vi "Feeding_OPEN_DOOR_ON_SCAN.vi"(7 "CYCLE DATA IN":T1, 8 "error in (no error)":errorcluster, 11 "raw scan code":string) -> (0 "error out":errorcluster, 2 "search valid ?":bool, 5 "CYCLE DATA OUT":T1)   [LabVIEW 2017]
uses:
  Controls/Feed_Cyc_Data.ctl
  <vilib>/Utility/file.llb/Read Delimited Spreadsheet (string).vi
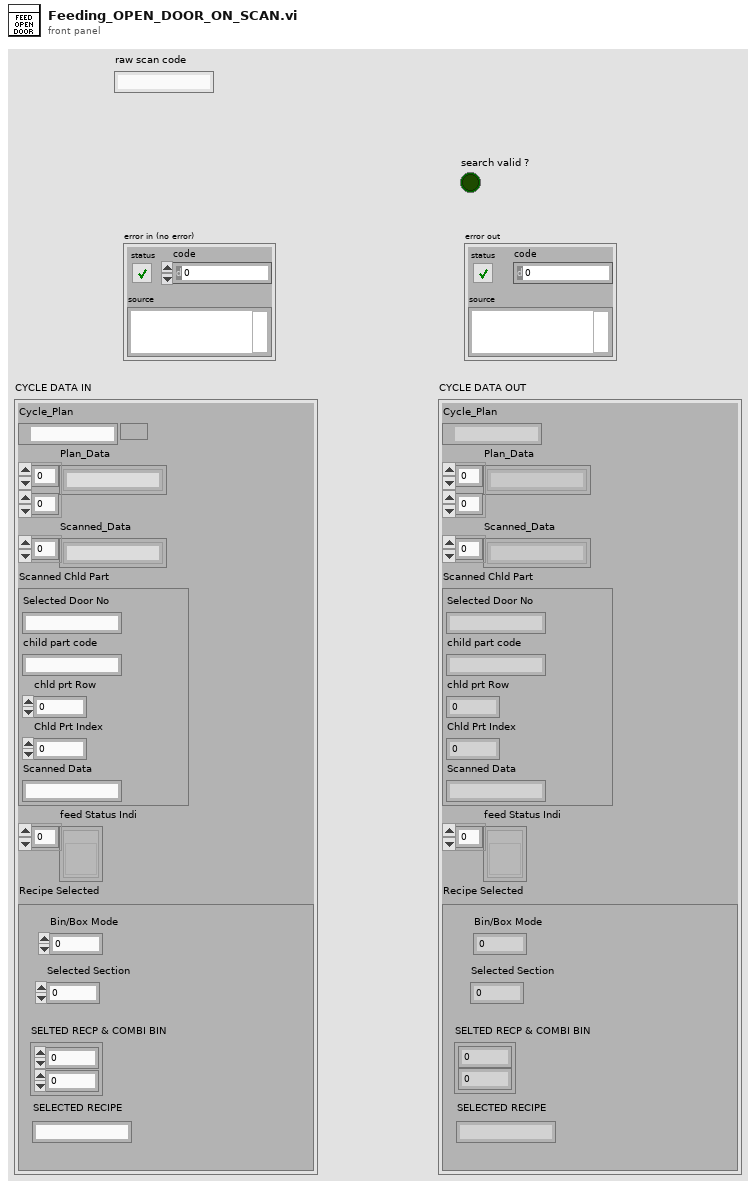
[diagram p1: front panel]
types:
  T1 = typedef "Feed_Cyc_Data.ctl" = cluster{"Cycle_Plan":path, "Plan_Data":string[][], "Scanned_Data":string[], "Scanned Chld Part":cluster{"Selected Door No":string, "child part code":string, "chld prt Row":i32, "Chld Prt Index":i32, "Scanned Data":string}, "feed Status Indi":refnum<vi>[], "Recipe Selected":cluster{"Bin/Box Mode":i32, "Selected Section":i32, "SELTED RECP & COMBI BIN":cluster{i32, i32}, "SELECTED RECIPE":string}}
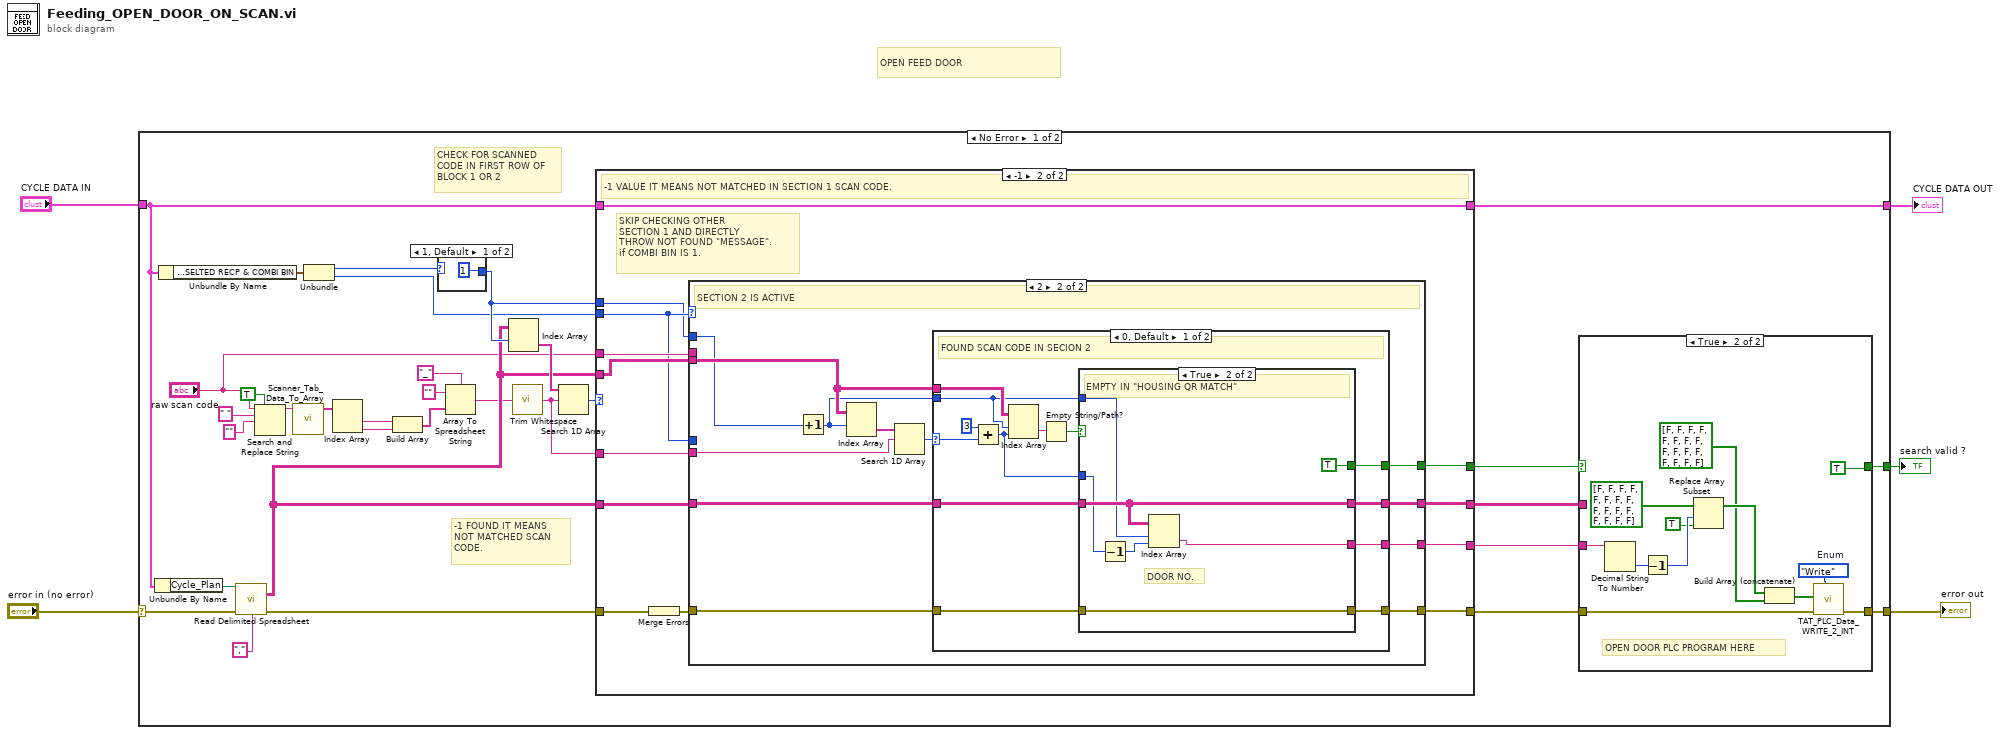
[diagram p0: block diagram]
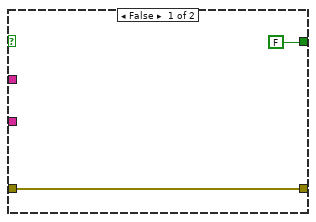
[diagram p2: hidden frame]
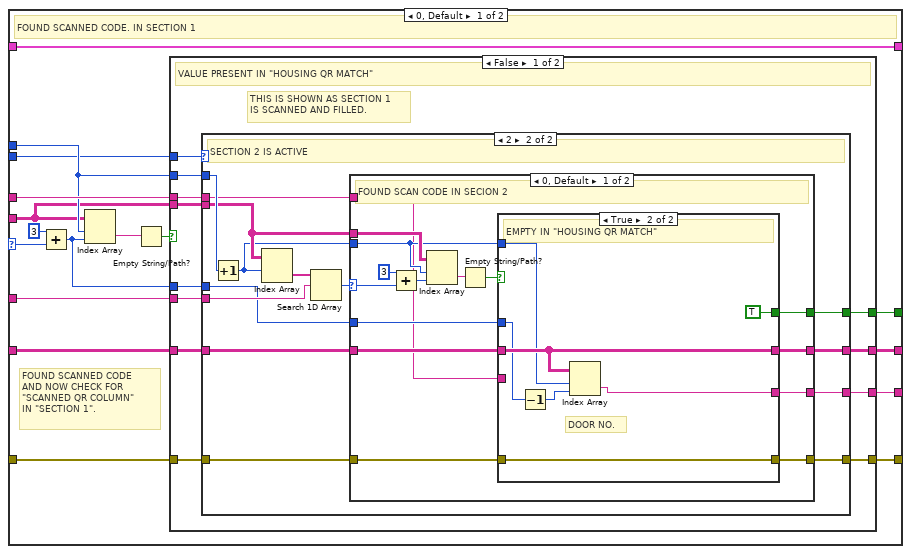
[diagram p3: hidden frame]
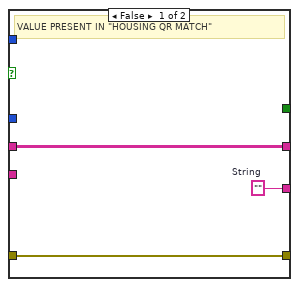
[diagram p5: hidden frame]
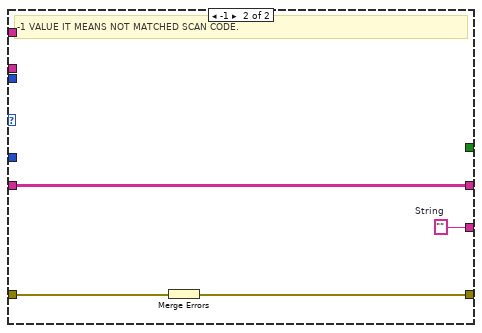
[diagram p6: hidden frame]
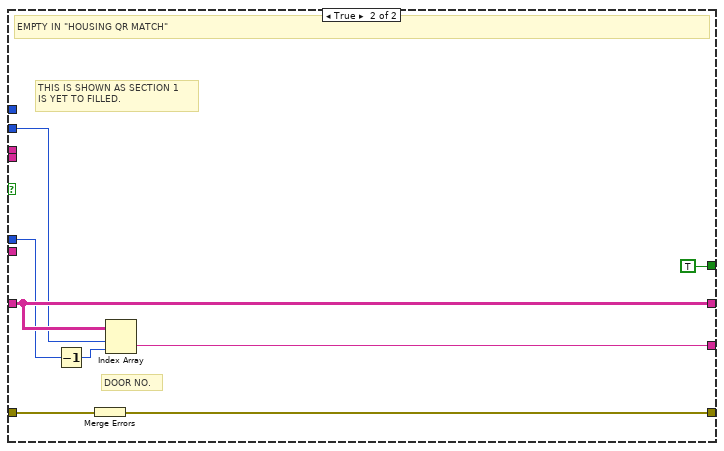
[diagram p7: hidden frame]
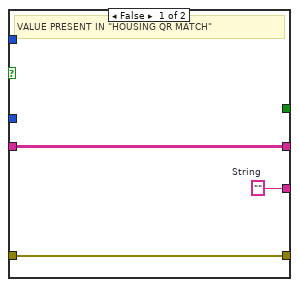
[diagram p9: hidden frame]
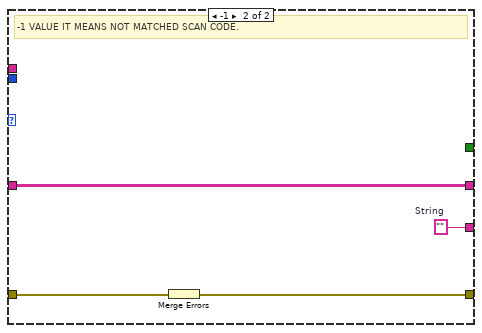
[diagram p10: hidden frame]
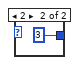
[diagram p11: hidden frame]
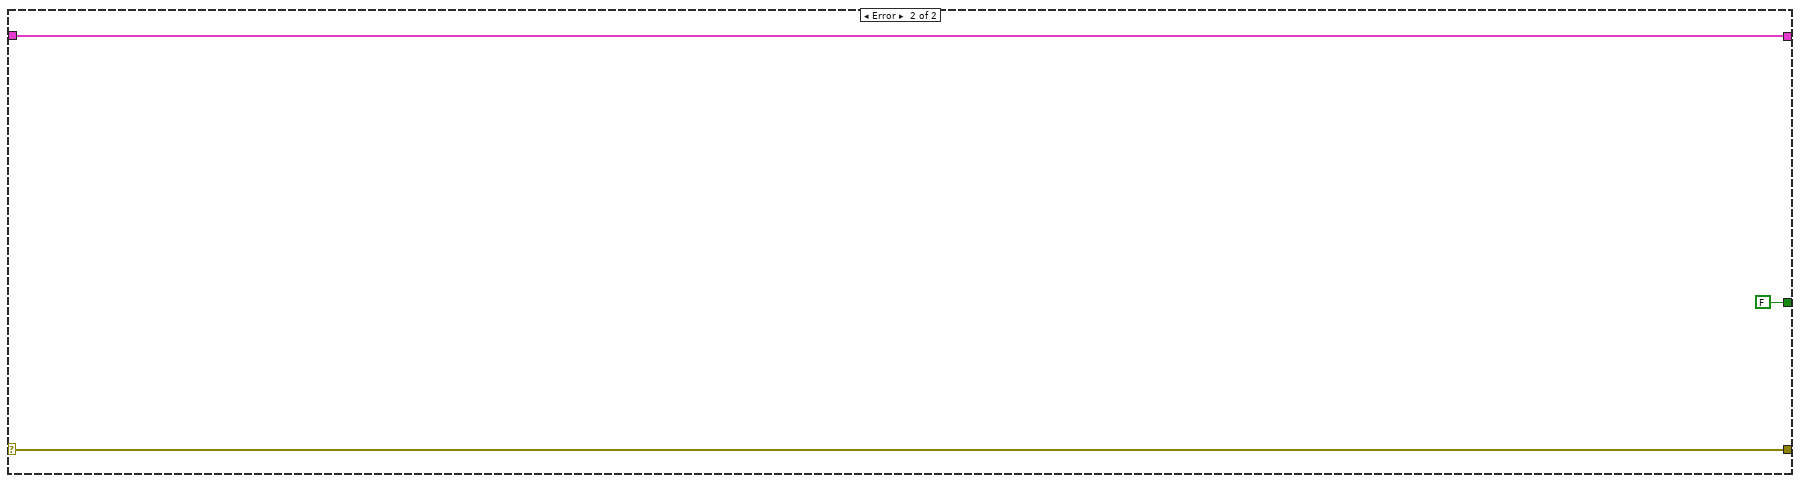
[diagram p12: hidden frame]
diagram:
  # "OPEN FEED DOOR"
  n1 = case shown="No Error" "error in (no error)" {
    selector: "error in (no error)" -> [w34 w192]
    tunnel: [w18 w192] -> w4
    tunnel: [w16 w191] -> w2
    tunnel: "CYCLE DATA IN" -> [w23 w191]
    tunnel: [w8 FALSE] -> w1
    frame No Error {
      # "-1 FOUND IT MEANS\nNOT MATCHED SCAN\nCODE."
      # "CHECK FOR SCANNED\nCODE IN FIRST ROW OF\nBLOCK 1 OR 2"
      n2 = Unbundle By Name(w23) -> ("Cycle_Plan"=w35:path)
      n3 = Unbundle By Name(w23) -> ("Recipe Selected.SELTED RECP & COMBI BIN"=w32:cluster{i32, i32})
      n4 = call-poly <vilib>:"Read Delimited Spreadsheet.vi"("file path (dialog if empty)"=w35, "error in (no error)"=w34, "delimiter (\\t)"=",") -> ("all rows"=w20:string[][], "error out"=w33:errorcluster)  [unwired: 7 in, 4 out]
      n5 = Search and Replace String(replace all?=TRUE, input string="raw scan code", search string=" ", replace string="") -> (result string=w30:string)  [unwired: 4 in, 3 out]
      n6 = call "Scanner_Tab_Data_To_Array.vi"("Scanner Data"=w30) -> ("Array"=w14:string[])  [unwired: 10 in]
      n7 = Unbundle(w32) -> (w31:i32, w19:i32)
      n8 = Index Array(array=w14) -> (element #1=w13:string, element #2=w12:string)  [unwired: 2 in]
      n9 = Build Array(w13, w12) -> (w11:string[])
      n10 = case shown="1, Default" w31 {
        tunnel: [1 3] -> w21
        frame 1, Default {
        }
        frame 2 {
        }
      }
      n11 = Array To Spreadsheet String(delimiter (Tab)="_", array=w11, 3:"") -> (spreadsheet string=w10:string)
      n12 = Index Array(array=w20, index (row)=w21) -> (element=w24:string[])  [unwired: 1 in]
      n13 = call <vilib>:"Trim Whitespace.vi"("string"=w10) -> ("trimmed string"=w6:string)  [unwired: 1 in]
      n14 = Search 1D Array(1D array=w24, element=w6) -> (index of element=w22:i32)  [unwired: 1 in]
      n15 = case shown="-1" w22 {
        selector: w22 -> [w67 _]
        tunnel: [w64 w142] -> w37
        tunnel: w33 -> [w68 w146]
        tunnel: [w61 w145] -> w16
        tunnel: w23 -> [w61 w145]
        tunnel: w20 -> [w55 w137]
        tunnel: w21 -> [w59 w134]
        tunnel: "raw scan code" -> [w62 w138]
        tunnel: w20 -> [w60 w144]
        tunnel: [w57 w140] -> w15
        tunnel: w19 -> [w56 w136]
        tunnel: w6 -> [w54 w135]
        tunnel: [w53 w139] -> w17
        tunnel: [w52 w141] -> w9
        frame 0, Default {
          # "FOUND SCANNED CODE\nAND NOW CHECK FOR\n\"SCANNED QR COLUMN\"\nIN \"SECTION 1\"."
          # "FOUND SCANNED CODE. IN SECTION 1"
          n16 = Add(x=3, y=w67) -> (x+y=w58:i32)
          n17 = Index Array(array=w55, index (row)=w59, index (col)=w58) -> (element=w65:string)
          n18 = Empty String/Path?(string/path=w65) -> (empty?=w63:bool)
          n19 = case shown="False" w63 {
            tunnel: w68 -> [w79 w133]
            tunnel: [w80 w132] -> w64
            tunnel: w62 -> [w71 _]
            tunnel: w60 -> [w76 w131]
            tunnel: w59 -> [w75 w129]
            tunnel: w58 -> [w73 w128]
            tunnel: [w77 w131] -> w57
            tunnel: w56 -> [w78 _]
            tunnel: w55 -> [w74 _]
            tunnel: w54 -> [w72 _]
            tunnel: [w70 TRUE] -> w53
            tunnel: [w69 w126] -> w52
            frame False {
              # "THIS IS SHOWN AS SECTION 1\nIS SCANNED AND FILLED."
              # "VALUE PRESENT IN \"HOUSING QR MATCH\""
              n20 = case shown="2" w78 {
                tunnel: [w82 w92] -> w80
                tunnel: w79 -> [w82 w96]
                tunnel: [w81 w91] -> w77
                tunnel: w76 -> [w81 w90]
                tunnel: w75 -> [_ w95]
                tunnel: w74 -> [_ w88]
                tunnel: w73 -> [_ w86]
                tunnel: w72 -> [_ w93]
                tunnel: w71 -> [_ w85]
                tunnel: [_ w84] -> w70
                tunnel: [_ w83] -> w69
                frame 1, Default {
                  # "ONLY SECTION 1"
                }
                frame 2 {
                  # "SECTION 2 IS ACTIVE"
                  n21 = Increment(x=w95) -> (x+1=w87:i32)
                  n22 = Index Array(array=w88, index (row)=w87) -> (element=w94:string[])  [unwired: 1 in]
                  n23 = Search 1D Array(1D array=w94, element=w93) -> (index of element=w89:i32)  [unwired: 1 in]
                  n24 = case shown="0, Default" w89 {
                    selector: w89 -> [w108 _]
                    tunnel: w96 -> [w111 w125]
                    tunnel: [w106 w124] -> w92
                    tunnel: [w103 w123] -> w91
                    tunnel: w90 -> [w102 w123]
                    tunnel: w88 -> [w107 _]
                    tunnel: w87 -> [w101 _]
                    tunnel: w86 -> [w100 _]
                    tunnel: w85 -> [w99 _]
                    tunnel: [w98 _] -> w84
                    tunnel: [w97 w122] -> w83
                    frame 0, Default {
                      # "FOUND SCAN CODE IN SECION 2"
                      n25 = Add(x=3, y=w108) -> (x+y=w110:i32)
                      n26 = Index Array(array=w107, index (row)=w101, index (col)=w110) -> (element=w105:string)
                      n27 = Empty String/Path?(string/path=w105) -> (empty?=w104:bool)
                      n28 = case shown="True" w104 {
                        tunnel: w111 -> [w113 w121]
                        tunnel: [w113 w121] -> w106
                        tunnel: [w114 w118] -> w103
                        tunnel: w102 -> [w114 w118]
                        tunnel: w101 -> [_ w117]
                        tunnel: w100 -> [_ w116]
                        tunnel: w99 -> [_ _]
                        tunnel: [_ TRUE] -> w98
                        tunnel: [w112 w115] -> w97
                        frame False {
                          w112 = ""  # String
                          # "VALUE PRESENT IN \"HOUSING QR MATCH\""
                        }
                        frame True {
                          # "DOOR NO."
                          # "EMPTY IN \"HOUSING QR MATCH\""
                          n29 = Decrement(x=w116) -> (x-1=w119:i32)
                          n30 = Index Array(array=w118, index (row)=w117, index (col)=w119) -> (element=w115:string)
                        }
                      }
                    }
                    frame -1 {
                      w122 = ""  # String
                      # "-1 VALUE IT MEANS NOT MATCHED SCAN CODE."
                      n31 = Merge Errors(w125) -> (w124:errorcluster)
                    }
                  }
                }
              }
            }
            frame True {
              # "DOOR NO."
              # "THIS IS SHOWN AS SECTION 1\nIS YET TO FILLED."
              # "EMPTY IN \"HOUSING QR MATCH\""
              n32 = Decrement(x=w128) -> (x-1=w127:i32)
              n33 = Merge Errors(w133) -> (w132:errorcluster)
              n34 = Index Array(array=w131, index (row)=w129, index (col)=w127) -> (element=w126:string)
            }
          }
        }
        frame -1 {
          # "SKIP CHECKING OTHER \nSECTION 1 AND DIRECTLY\nTHROW NOT FOUND \"MESSAGE\". \nif COMBI BIN IS 1."
          # "-1 VALUE IT MEANS NOT MATCHED IN SECTION 1 SCAN CODE."
          n35 = Merge Errors(w146) -> (w143:errorcluster)
          n36 = case shown="2" w136 {
            tunnel: [w148 w157] -> w142
            tunnel: w143 -> [w148 w160]
            tunnel: [w147 w156] -> w140
            tunnel: w144 -> [w147 w155]
            tunnel: w137 -> [_ w153]
            tunnel: w136 -> [_ _]
            tunnel: w135 -> [_ w158]
            tunnel: w138 -> [_ _]
            tunnel: [_ w151] -> w139
            tunnel: [_ w150] -> w141
            tunnel: w134 -> [_ w149]
            frame 1, Default {
              # "ONLY SECTION 1"
            }
            frame 2 {
              # "SECTION 2 IS ACTIVE"
              n37 = Increment(x=w149) -> (x+1=w152:i32)
              n38 = Index Array(array=w153, index (row)=w152) -> (element=w159:string[])  [unwired: 1 in]
              n39 = Search 1D Array(1D array=w159, element=w158) -> (index of element=w154:i32)  [unwired: 1 in]
              n40 = case shown="0, Default" w154 {
                selector: w154 -> [w171 _]
                tunnel: w160 -> [w173 w187]
                tunnel: [w169 w186] -> w157
                tunnel: [w166 w185] -> w156
                tunnel: w155 -> [w165 w185]
                tunnel: w153 -> [w170 _]
                tunnel: w152 -> [w164 _]
                tunnel: [w163 _] -> w151
                tunnel: [w162 w184] -> w150
                frame 0, Default {
                  # "FOUND SCAN CODE IN SECION 2"
                  n41 = Add(x=3, y=w171) -> (x+y=w161:i32)
                  n42 = Index Array(array=w170, index (row)=w164, index (col)=w161) -> (element=w168:string)
                  n43 = Empty String/Path?(string/path=w168) -> (empty?=w167:bool)
                  n44 = case shown="True" w167 {
                    tunnel: w173 -> [w175 w183]
                    tunnel: [w175 w183] -> w169
                    tunnel: [w176 w180] -> w166
                    tunnel: w165 -> [w176 w180]
                    tunnel: w164 -> [_ w179]
                    tunnel: w161 -> [_ w178]
                    tunnel: [_ TRUE] -> w163
                    tunnel: [w174 w177] -> w162
                    frame False {
                      w174 = ""  # String
                      # "VALUE PRESENT IN \"HOUSING QR MATCH\""
                    }
                    frame True {
                      # "DOOR NO."
                      # "EMPTY IN \"HOUSING QR MATCH\""
                      n45 = Decrement(x=w178) -> (x-1=w181:i32)
                      n46 = Index Array(array=w180, index (row)=w179, index (col)=w181) -> (element=w177:string)
                    }
                  }
                }
                frame -1 {
                  w184 = ""  # String
                  # "-1 VALUE IT MEANS NOT MATCHED SCAN CODE."
                  n47 = Merge Errors(w187) -> (w186:errorcluster)
                }
              }
            }
          }
        }
      }
      n48 = case shown="True" w17 {
        tunnel: w37 -> [w39 w45]
        tunnel: [w39 w44] -> w18
        tunnel: w15 -> [_ _]
        tunnel: w9 -> [_ w51]
        tunnel: [FALSE TRUE] -> w8
        frame False {
        }
        frame True {
          w50 = enum16{"Read", "Write"}."Write"  # Enum
          # "OPEN DOOR PLC PROGRAM HERE"
          n49 = Decimal String To Number(string=w51) -> (number=w46:i32)  [unwired: 2 in, 1 out]
          n50 = Decrement(x=w46) -> (x-1=w48:i32)
          n51 = Replace Array Subset(array=bool[] [FALSE, FALSE, FALSE, FALSE, FALSE, FALSE, FALSE, FALSE, FALSE, FALSE, FALSE, FALSE, FALSE, FALSE, FALSE, FALSE], new element=TRUE, index=w48) -> (w42:bool[])
          n52 = Build Array (concatenate)(w42, bool[] [FALSE, FALSE, FALSE, FALSE, FALSE, FALSE, FALSE, FALSE, FALSE, FALSE, FALSE, FALSE, FALSE, FALSE, FALSE, FALSE]) -> (w43:bool[])
          n53 = call "TAT_PLC_Data_WRITE_2_INT.vi"("Enum"=w50, "error in (no error)"=w45, "Array"=w43) -> ("error out"=w44:errorcluster)  [unwired: 7 in, 1 out]
        }
      }
    }
    frame Error {
    }
  }
  "error out" <- w4
  "CYCLE DATA OUT" <- w2
  "search valid ?" <- w1
